vi "标样核查.vi"(11 "标样核查配置":T1={"数据保存间隔"=1.0, "水温标样值"=0.0, "pH标样值"=0.0, "溶解氧标样值"=0.0, "电导率标样值"=0.0, "浊度标样值"=0.0}) -> ()   [LabVIEW 2016, in "斯坦道多参数.lvlib"]
panel:
  out "运行状态":u16(ring) items=["空闲", "水样测试", "标样核查"]
  out "seconds since 1Jan1904":timestamp
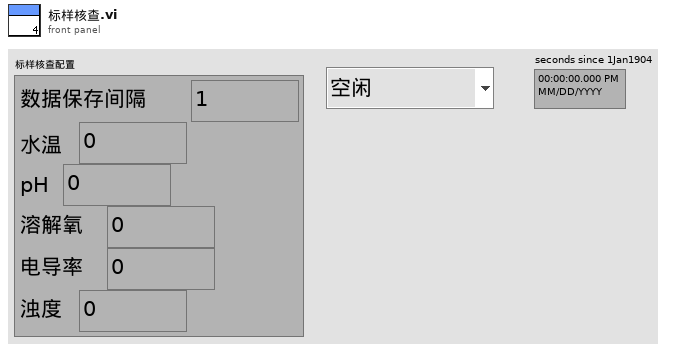
[diagram p1: front panel]
types:
  T1 = cluster{"数据保存间隔":dbl, "水温标样值":dbl, "pH标样值":dbl, "溶解氧标样值":dbl, "电导率标样值":dbl, "浊度标样值":dbl}
  T2 = cluster{"ph":bool, "DO":bool, "Cond":bool, "Turb":bool, "叶绿素a":bool, "藻密度":bool, "ORP":bool}
  T3 = cluster{"因子编码":string, "单位":string, "标样参考值":sgl, "水样数据时间":timestamp, "水样实测值":sgl, "水样数据标识":string, "探头温度":sgl}
  T4 = typedef "LVDateTimeRec.ctl" = cluster{"秒数的小数部分":dbl, "秒":i32, "分":i32, "时":i32, "日":i32, "月":i32, "年":i32, "天数（周）":i32, "天数（年）":i32, "DST":i32}
  T5 = cluster{"温度测量值":sgl, "DO%":sgl, "DOmg/L":sgl, "温度偏移修正值":sgl}
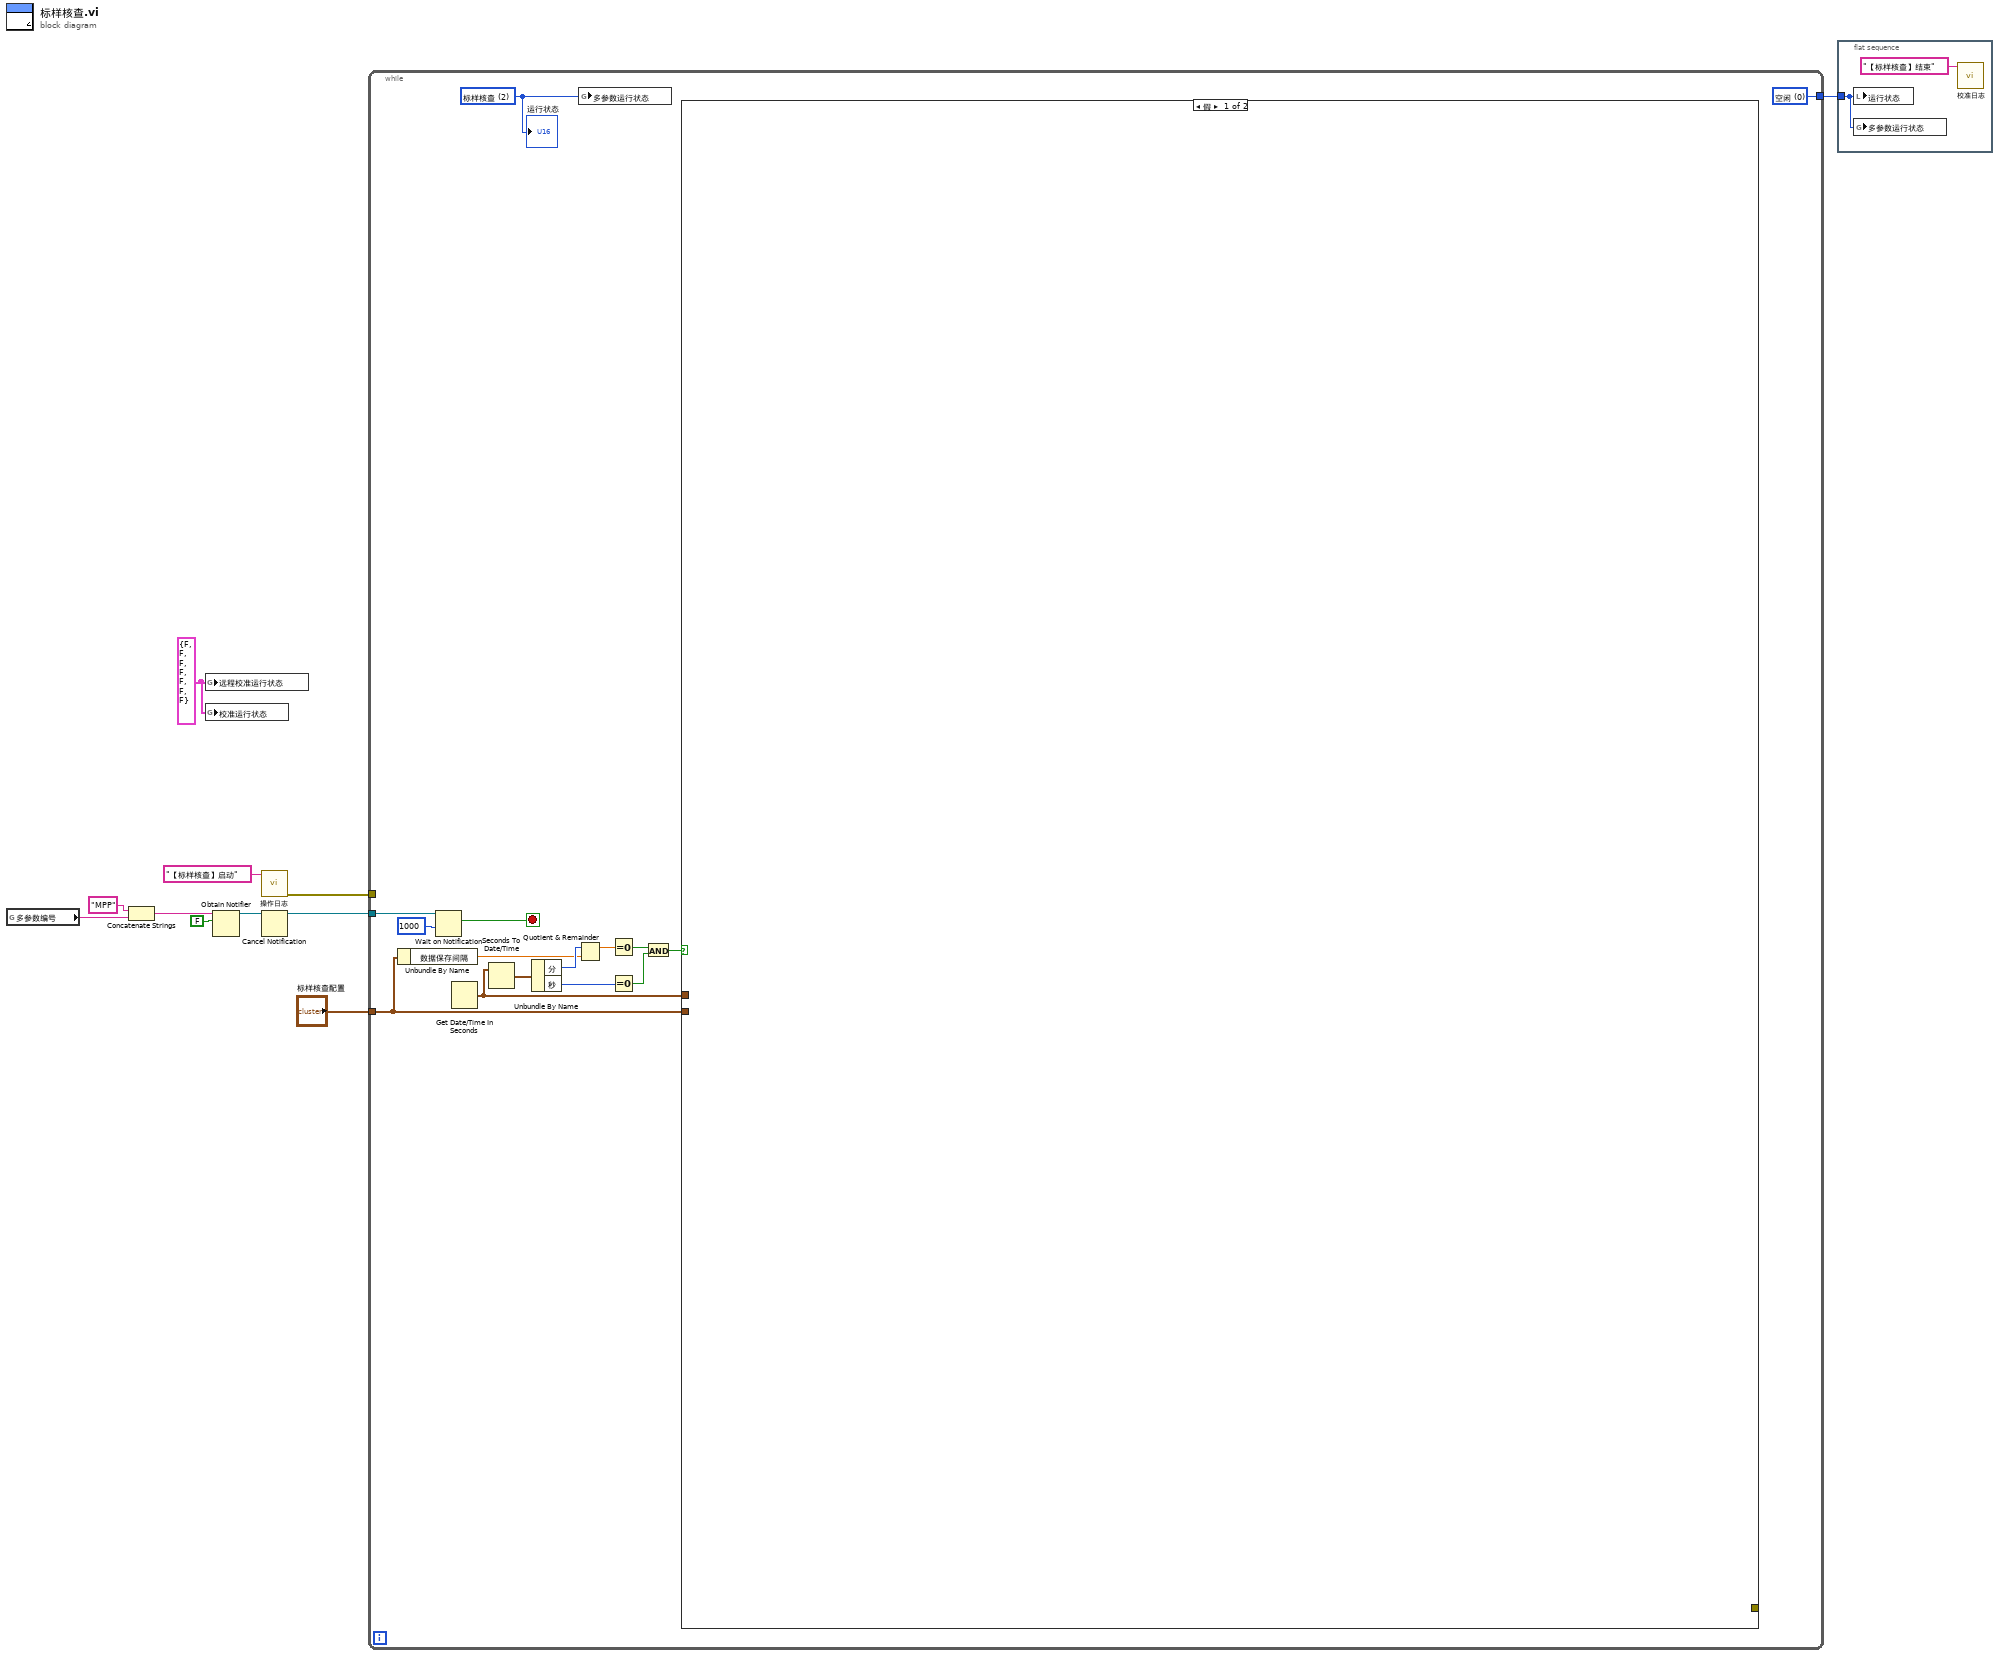
[diagram p0: block diagram]
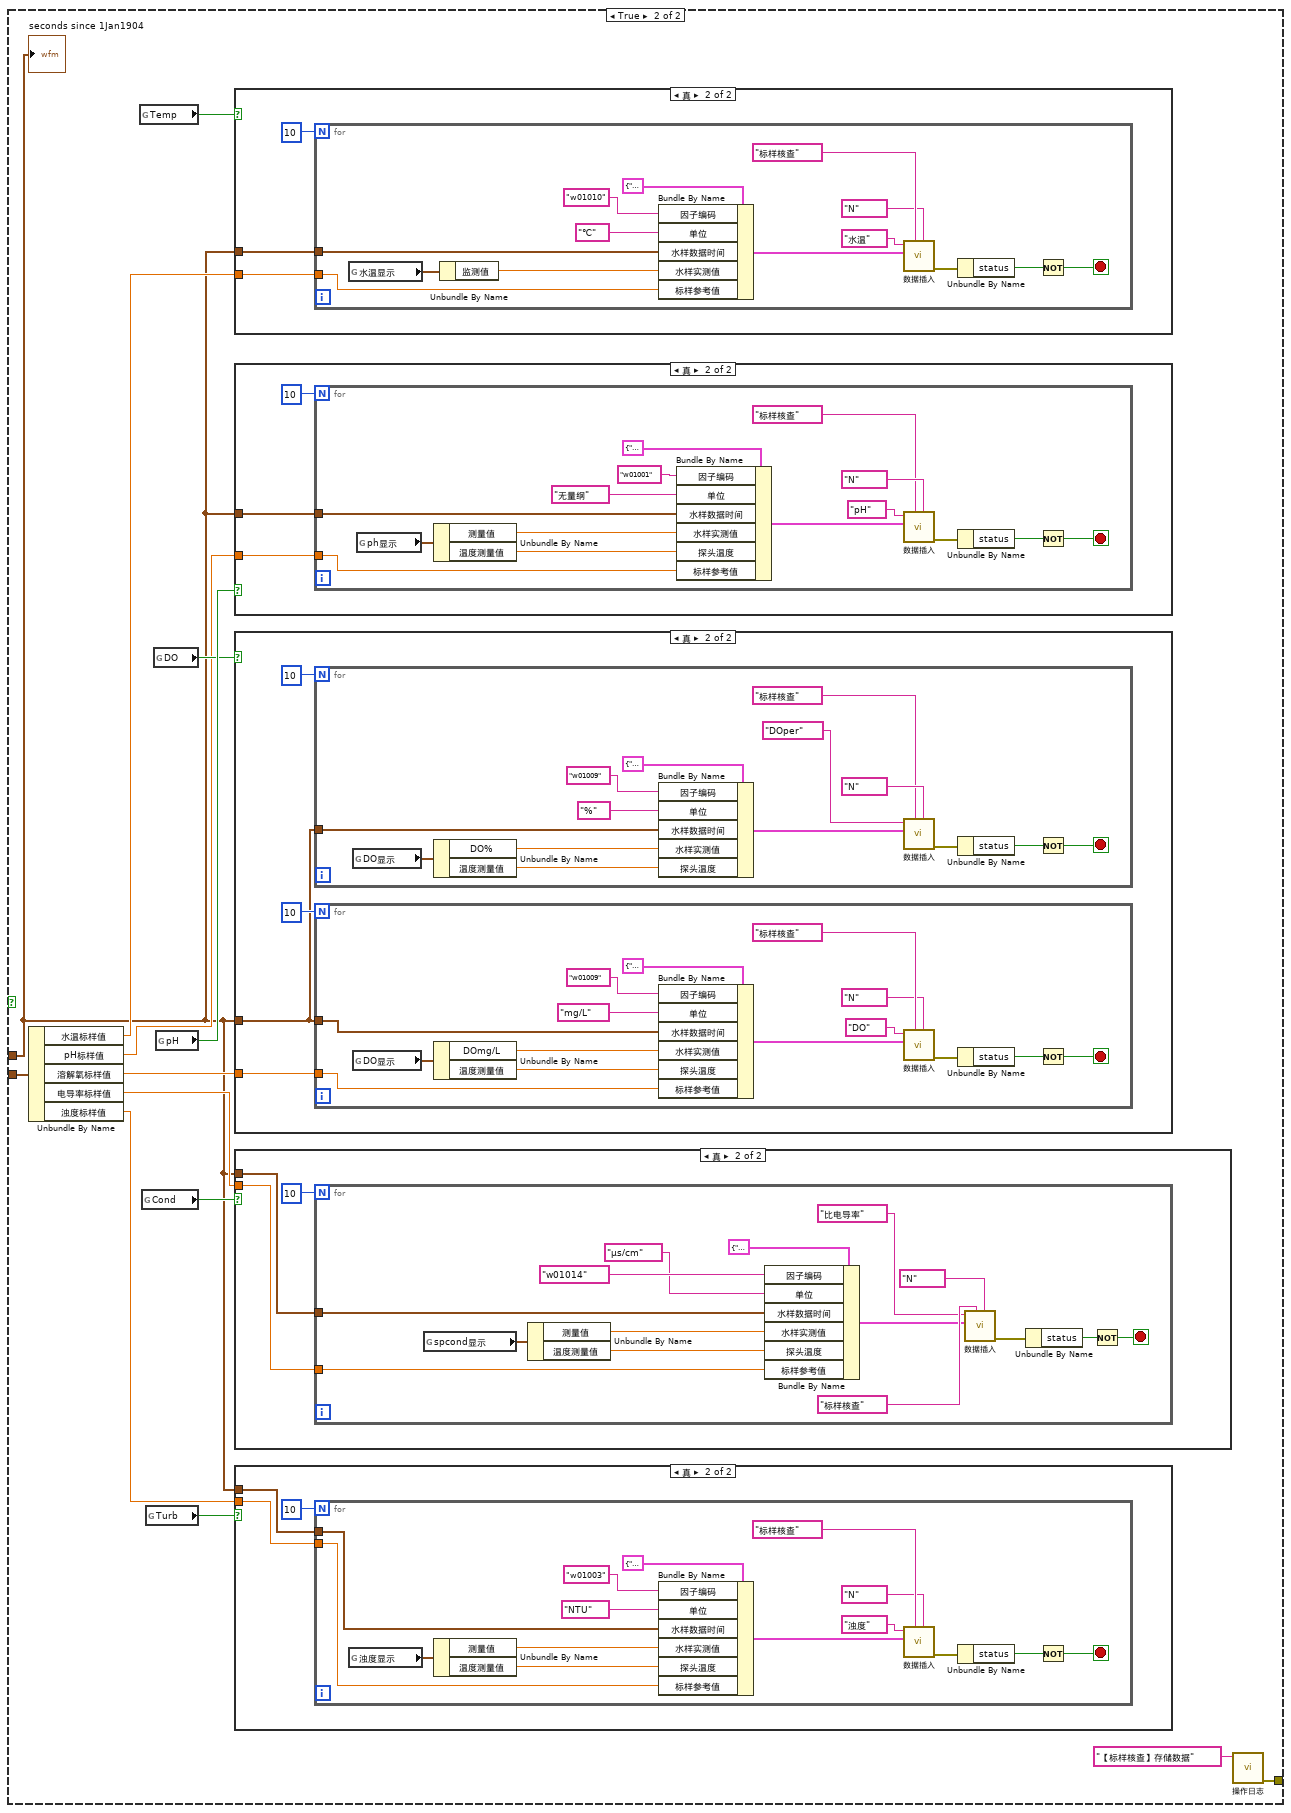
[diagram p2: hidden frame]
diagram:
  w1 = T2 {"ph"=FALSE, "DO"=FALSE, "Cond"=FALSE, "Turb"=FALSE, "叶绿素a"=FALSE, "藻密度"=FALSE, "ORP"=FALSE} ("校准运行状态")
  n1 = global read "多参数全局变量.vi" "多参数编号"() -> (w4:string)
  n2 = Concatenate Strings("MPP" ("名称（未命名）"), w4) -> (w5:string)
  n3 = global write "多参数全局变量.vi" "远程校准运行状态"(w1) -> ()
  n4 = global write "多参数全局变量.vi" "校准运行状态"(w1) -> ()
  n5 = Obtain Notifier(name (unnamed)=w5, notification data type=FALSE) -> (notifier out=w8:refnum<notifier>)  [unwired: 2 in, 2 out]
  n6 = call "操作日志.vi"("日志信息"="【标样核查】启动") -> ("error out"=w2:errorcluster)  [unwired: 10 in]
  n7 = Cancel Notification(0:w8) -> (8:w7:refnum<notifier>)  [unwired: 1 in, 2 out]
  n8 = while {
    tunnel: "标样核查配置" -> [w22]
    tunnel: [w16] -> w6
    tunnel: w7 -> [w15]
    tunnel: w2 -> [_]
    stop <- w13 stop-if-true
    w16 = u16 0 items=["空闲", "水样测试", "标样核查"] ("多参数运行状态")
    w12 = u16 2 items=["空闲", "水样测试", "标样核查"] ("多参数运行状态")
    n9 = Unbundle By Name(w22) -> ("数据保存间隔"=w20:dbl)
    n10 = Wait on Notification(notifier=w15, timeout in ms (-1)=1000 ("超时毫秒(-1)")) -> (notification=w13:bool)  [unwired: 2 in, 3 out]
    n11 = Get Date/Time In Seconds() -> (seconds since 1Jan1904=w17:timestamp)
    n12 = Seconds To Date/Time(time stamp (now)=w17) -> (date time rec=w26:T4)  [unwired: 1 in]
    n13 = Unbundle By Name(w26) -> ("分"=w21:i32, "秒"=w25:i32)
    n14 = Quotient & Remainder(x=w21, y=w20) -> (x-y*floor(x/y)=w19:dbl)  [unwired: 1 out]
    n15 = global write "多参数全局变量.vi" "多参数运行状态"(w12) -> ()
    n16 = Equal To 0?(x=w19) -> (x = 0?=w18:bool)
    n17 = Equal To 0?(x=w25) -> (x = 0?=w24:bool)
    n18 = And(x=w18, y=w24) -> (x .and. y?=w23:bool)
    n19 = case shown="假" w23 {
      tunnel: w22 -> [_ w35]
      tunnel: w17 -> [_ w27]
      tunnel: [_ w28] -> _
      frame False {
      }
      frame True {
        n20 = Unbundle By Name(w35) -> ("水温标样值"=w34:dbl, "pH标样值"=w33:dbl, "溶解氧标样值"=w32:dbl, "电导率标样值"=w31:dbl, "浊度标样值"=w30:dbl)
        n21 = global read "断电保存变量.vi" "Temp"() -> (w40:bool)
        n22 = global read "断电保存变量.vi" "Cond"() -> (w37:bool)
        n23 = global read "断电保存变量.vi" "Turb"() -> (w36:bool)
        n24 = global read "断电保存变量.vi" "DO"() -> (w38:bool)
        n25 = global read "断电保存变量.vi" "pH"() -> (w39:bool)
        n26 = case shown="真" w40 {
          tunnel: w34 -> [_ w130]
          tunnel: w27 -> [_ w129]
          frame False {
          }
          frame True {
            n27 = for {
              N: 10 -> [_]
              tunnel: w130 -> [w137]
              tunnel: w129 -> [w134]
              stop <- w131 stop-if-true
              n28 = global read "多参数全局变量.vi" "水温显示"() -> (w136:cluster{"CH":u16, "监测值":dbl, "温度偏移修正值":sgl})
              n29 = Unbundle By Name(w136) -> ("监测值"=w135:dbl)
              n30 = Bundle By Name(cluster=T3 {"因子编码"="w01003", "单位"="无量纲", "标样参考值"=0.0, "水样数据时间"=timestamp(0 s since 1904-01-01), "水样实测值"=0.0, "水样数据标识"="N", "探头温度"=0.0} ("data in"), "因子编码"="w01010", "单位"="℃", "水样数据时间"=w134, "水样实测值"=w135, "标样参考值"=w137) -> (w143:T3)
              n31 = call "数据插入.vi"("数据标记表"="N", "测量模式"="标样核查", "data in"=w143, "table输入"="水温") -> ("error out"=w133:errorcluster)  [unwired: 7 in]
              n32 = Unbundle By Name(w133) -> ("status"=w132:bool)
              n33 = Not(x=w132) -> (.not. x?=w131:bool)
            }
          }
        }
        n34 = case shown="真" w39 {
          tunnel: w33 -> [_ w112]
          tunnel: w27 -> [_ w110]
          frame False {
          }
          frame True {
            n35 = for {
              N: 10 -> [_]
              tunnel: w112 -> [w120]
              tunnel: w110 -> [w113]
              stop <- w114 stop-if-true
              n36 = global read "多参数全局变量.vi" "ph显示"() -> (w119:cluster{"温度测量值":sgl, "测量值":sgl, "温度偏移修正值":sgl})
              n37 = Unbundle By Name(w119) -> ("测量值"=w118:sgl, "温度测量值"=w117:sgl)
              n38 = Bundle By Name(cluster=T3 {"因子编码"="w01003", "单位"="无量纲", "标样参考值"=0.0, "水样数据时间"=timestamp(0 s since 1904-01-01), "水样实测值"=0.0, "水样数据标识"="N", "探头温度"=0.0} ("data in"), "因子编码"="w01001", "单位"="无量纲", "水样数据时间"=w113, "水样实测值"=w118, "探头温度"=w117, "标样参考值"=w120) -> (w125:T3)
              n39 = call "数据插入.vi"("数据标记表"="N", "测量模式"="标样核查", "data in"=w125, "table输入"="pH") -> ("error out"=w116:errorcluster)  [unwired: 7 in]
              n40 = Unbundle By Name(w116) -> ("status"=w115:bool)
              n41 = Not(x=w115) -> (.not. x?=w114:bool)
            }
          }
        }
        n42 = case shown="真" w38 {
          tunnel: w32 -> [_ w80]
          tunnel: w27 -> [_ w77]
          frame False {
          }
          frame True {
            n43 = for {
              N: 10 -> [_]
              tunnel: w77 -> [w81]
              stop <- w82 stop-if-true
              n44 = global read "多参数全局变量.vi" "DO显示"() -> (w85:T5)
              n45 = Unbundle By Name(w85) -> ("DO%"=w89:sgl, "温度测量值"=w87:sgl)
              n46 = Bundle By Name(cluster=T3 {"因子编码"="w01003", "单位"="无量纲", "标样参考值"=0.0, "水样数据时间"=timestamp(0 s since 1904-01-01), "水样实测值"=0.0, "水样数据标识"="N", "探头温度"=0.0} ("data in"), "因子编码"="w01009", "单位"="%", "水样数据时间"=w81, "水样实测值"=w89, "探头温度"=w87) -> (w86:T3)
              n47 = call "数据插入.vi"("数据标记表"="N", "测量模式"="标样核查", "data in"=w86, "table输入"="DOper") -> ("error out"=w84:errorcluster)  [unwired: 7 in]
              n48 = Unbundle By Name(w84) -> ("status"=w83:bool)
              n49 = Not(x=w83) -> (.not. x?=w82:bool)
            }
            n50 = for {
              N: 10 -> [_]
              tunnel: w80 -> [w100]
              tunnel: w77 -> [w95]
              stop <- w96 stop-if-true
              n51 = global read "多参数全局变量.vi" "DO显示"() -> (w99:T5)
              n52 = Unbundle By Name(w99) -> ("DOmg/L"=w107:sgl, "温度测量值"=w109:sgl)
              n53 = Bundle By Name(cluster=T3 {"因子编码"="w01003", "单位"="无量纲", "标样参考值"=0.0, "水样数据时间"=timestamp(0 s since 1904-01-01), "水样实测值"=0.0, "水样数据标识"="N", "探头温度"=0.0} ("data in"), "因子编码"="w01009", "单位"="mg/L", "水样数据时间"=w95, "水样实测值"=w107, "探头温度"=w109, "标样参考值"=w100) -> (w106:T3)
              n54 = call "数据插入.vi"("数据标记表"="N", "测量模式"="标样核查", "data in"=w106, "table输入"="DO") -> ("error out"=w98:errorcluster)  [unwired: 7 in]
              n55 = Unbundle By Name(w98) -> ("status"=w97:bool)
              n56 = Not(x=w97) -> (.not. x?=w96:bool)
            }
          }
        }
        n57 = case shown="真" w37 {
          tunnel: w31 -> [_ w61]
          tunnel: w27 -> [_ w59]
          frame False {
          }
          frame True {
            n58 = for {
              N: 10 -> [_]
              tunnel: w61 -> [w70]
              tunnel: w59 -> [w63]
              stop <- w64 stop-if-true
              n59 = global read "多参数全局变量.vi" "spcond显示"() -> (w69:cluster{"温度测量值":sgl, "测量值":sgl, "温度偏移修正值":sgl})
              n60 = Unbundle By Name(w69) -> ("测量值"=w68:sgl, "温度测量值"=w67:sgl)
              n61 = Bundle By Name(cluster=T3 {"因子编码"="w01003", "单位"="无量纲", "标样参考值"=0.0, "水样数据时间"=timestamp(0 s since 1904-01-01), "水样实测值"=0.0, "水样数据标识"="N", "探头温度"=0.0} ("data in"), "因子编码"="w01014", "单位"="μs/cm", "水样数据时间"=w63, "水样实测值"=w68, "探头温度"=w67, "标样参考值"=w70) -> (w74:T3)
              n62 = call "数据插入.vi"("数据标记表"="N", "测量模式"="标样核查", "data in"=w74, "table输入"="比电导率") -> ("error out"=w66:errorcluster)  [unwired: 7 in]
              n63 = Unbundle By Name(w66) -> ("status"=w65:bool)
              n64 = Not(x=w65) -> (.not. x?=w64:bool)
            }
          }
        }
        n65 = case shown="真" w36 {
          tunnel: w30 -> [_ w43]
          tunnel: w27 -> [_ w41]
          frame False {
          }
          frame True {
            n66 = for {
              N: 10 -> [_]
              tunnel: w43 -> [w51]
              tunnel: w41 -> [w44]
              stop <- w45 stop-if-true
              n67 = global read "多参数全局变量.vi" "浊度显示"() -> (w50:cluster{"温度测量值":sgl, "测量值":sgl, "温度偏移修正值":sgl})
              n68 = Unbundle By Name(w50) -> ("测量值"=w49:sgl, "温度测量值"=w48:sgl)
              n69 = Bundle By Name(cluster=T3 {"因子编码"="w01003", "单位"="无量纲", "标样参考值"=0.0, "水样数据时间"=timestamp(0 s since 1904-01-01), "水样实测值"=0.0, "水样数据标识"="N", "探头温度"=0.0} ("data in"), "因子编码"="w01003", "单位"="NTU", "水样数据时间"=w44, "水样实测值"=w49, "探头温度"=w48, "标样参考值"=w51) -> (w57:T3)
              n70 = call "数据插入.vi"("数据标记表"="N", "测量模式"="标样核查", "data in"=w57, "table输入"="浊度") -> ("error out"=w47:errorcluster)  [unwired: 7 in]
              n71 = Unbundle By Name(w47) -> ("status"=w46:bool)
              n72 = Not(x=w46) -> (.not. x?=w45:bool)
            }
          }
        }
        n73 = call "操作日志.vi"("日志信息"="【标样核查】存储数据") -> ("error out"=w28:errorcluster)  [unwired: 10 in]
        "seconds since 1Jan1904" <- w27
      }
    }
    "运行状态" <- w12
  }
  n74 = flat-sequence {
    tunnel: w6 -> [w146]
    frame #0 {
      n75 = local write "运行状态"(w146) -> ()
      n76 = global write "多参数全局变量.vi" "多参数运行状态"(w146) -> ()
      n77 = call "校准日志.vi"("日志信息"="【标样核查】结束") -> ()  [unwired: 10 in, 1 out]
    }
  }
